vi "Time stamp to time string.vi"(8 "error in (no error)":errorcluster, 10 "Time Stamp":timestamp, 11 "OLE DB Timestamp in":refnum<class "OLE DB Timestamp.lvclass">) -> (0 "error out":errorcluster, 2 "String":string, 3 "OLE DB Timestamp out":refnum<class "OLE DB Timestamp.lvclass">)   [LabVIEW 2020, in "Basic Columns.lvlib" / "OLE DB Timestamp.lvclass"]
uses:
  OLE DB Timestamp.lvclass
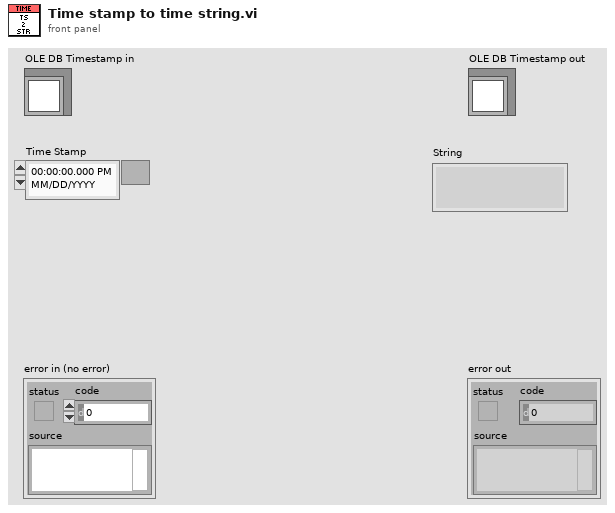
[diagram p1: front panel]
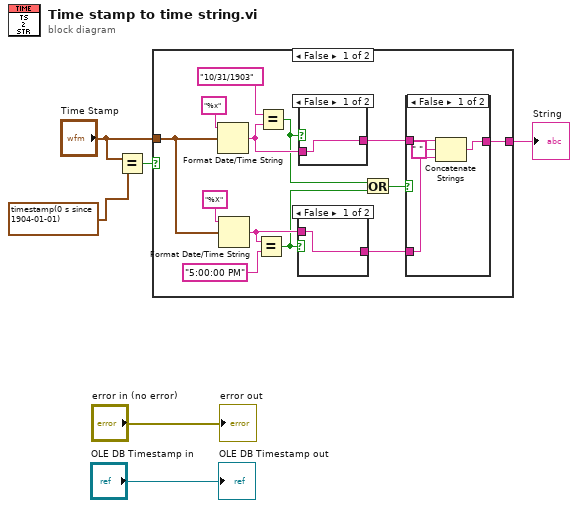
[diagram p0: block diagram]
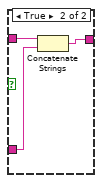
[diagram p2: hidden frame]
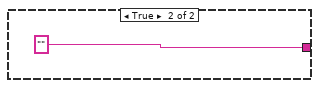
[diagram p5: hidden frame]
diagram:
  n1 = Equal?(x="Time Stamp", y=timestamp(0 s since 1904-01-01) ("Time Stamp")) -> (x = y?=w2:bool)
  n2 = case shown="False" w2 {
    tunnel: [w7 "" ("date/time string")] -> w1
    tunnel: "Time Stamp" -> [w17 _]
    frame False {
      n3 = Format Date/Time String(time format string (%c)="%x" ("format string"), seconds (now)=w17) -> (date/time string=w15:string)  [unwired: 1 in]
      n4 = Format Date/Time String(time format string (%c)="%X" ("format string"), seconds (now)=w17) -> (date/time string=w16:string)  [unwired: 1 in]
      n5 = Equal?(x=w16, y="5:00:00 PM") -> (x = y?=w10:bool)
      n6 = Equal?(x="10/31/1903", y=w15) -> (x = y?=w11:bool)
      n7 = case shown="False" w10 {
        tunnel: w16 -> [w28 _]
        tunnel: [w28 _] -> w8
        frame False {
        }
        frame True {
        }
      }
      n8 = case shown="False" w11 {
        tunnel: w15 -> [w27 _]
        tunnel: [w27 _] -> w9
        frame False {
        }
        frame True {
        }
      }
      n9 = Or(x=w11, y=w10) -> (x .or. y?=w12:bool)
      n10 = case shown="False" w12 {
        tunnel: w9 -> [w23 w25]
        tunnel: w8 -> [w22 w24]
        tunnel: [w20 w26] -> w7
        frame False {
          n11 = Concatenate Strings(w23, " " ("string"), w22) -> (w20:string)
        }
        frame True {
          n12 = Concatenate Strings(w25, w24) -> (w26:string)
        }
      }
    }
    frame True {
    }
  }
  "String" <- w1
  "error out" <- "error in (no error)"
  "OLE DB Timestamp out" <- "OLE DB Timestamp in"
